vi "controlRelativeTargetPosition.vi"() -> ()   [LabVIEW 2015, in "AMC_VIs.lvlib"]
uses:
  AMC_VIs.lvlib
panel:
  out "error out":errorcluster
  in  "error in":errorcluster
  in  "deviceAddress":string
  in  "connection ID":refnum<k5>
  out "New Target Position [nm]":dbl
  in  "MoveRelDistance [nm]":dbl format="%#_13g"
  in  "axis":i32
  in  "MoveRelBackward?":bool=TRUE
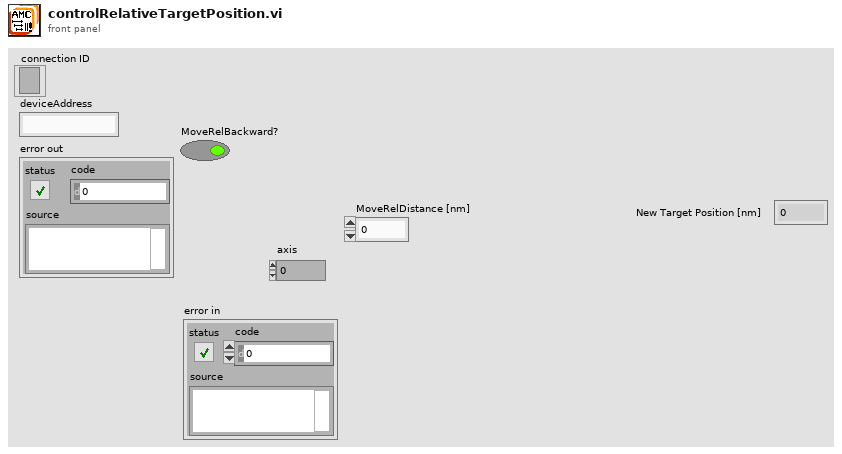
[diagram p1: front panel]
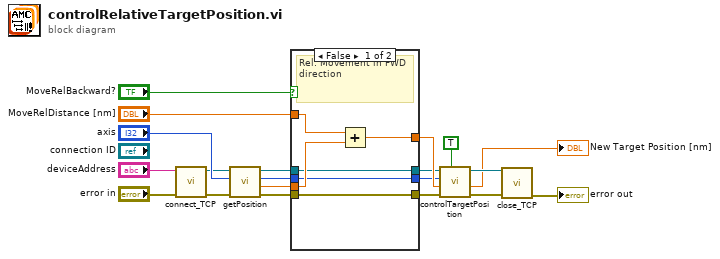
[diagram p0: block diagram]
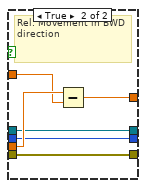
[diagram p2: hidden frame]
diagram:
  n1 = call "connect_TCP.vi"("error in"="error in", "deviceAddress"="deviceAddress") -> ("error ECC_connect"=w7:errorcluster, "connection ID"=w5:refnum<k5>)  [unwired: 4 in]
  n2 = call "getPosition.vi"("error in"=w7, "axis"="axis", "connection ID"=w5) -> ("error out"=w10:errorcluster, "position"=w19:dbl, "axis_out"=w15:i32, "connection ID"=w2:refnum<k5>)  [unwired: 5 in]
  n3 = case shown="False" "MoveRelBackward?" {
    tunnel: w19 -> [w25 w32]
    tunnel: "MoveRelDistance [nm]" -> [w26 w31]
    tunnel: [w24 w29] -> w16
    tunnel: w15 -> [w23 w30]
    tunnel: [w23 w30] -> w14
    tunnel: w10 -> [w22 w28]
    tunnel: [w22 w28] -> w9
    tunnel: w2 -> [w21 w27]
    tunnel: [w21 w27] -> w1
    frame False {
      # "Rel. Movement in FWD direction"
      n4 = Add(x=w26, y=w25) -> (x+y=w24:dbl)
    }
    frame True {
      # "Rel. Movement in BWD direction"
      n5 = Subtract(x=w32, y=w31) -> (x-y=w29:dbl)
    }
  }
  n6 = call "controlTargetPosition.vi"("Set"=TRUE, "error in"=w9, "Target Position [nm/µdeg]"=w16, "axis in"=w14, "connection ID"=w1) -> ("error out"=w13:errorcluster, "Target Position out"=→"New Target Position [nm]":dbl, "connection ID"=w12:refnum<k5>)  [unwired: 3 in, 1 out]
  n7 = call "close_TCP.vi"("error in"=w13, "connection ID"=w12) -> ("error out"=→"error out":errorcluster)  [unwired: 5 in]
